vi "comm trail.vi"() -> ()   [LabVIEW 2017]
uses:
  <vilib>/NI/Modbus Library/API/Wrapper/Create TCP Master.vi
  <vilib>/NI/Modbus Library/API/master/Modbus Master.lvclass
  <vilib>/NI/Modbus Library/API/Wrapper/API Main.lvlib
panel:
  out "*(type *) &x":sgl
  out "*(type *) &x 2":sgl
  out "Converted Array":sgl[](array[numeric])
  out "register values 2":u16[](array[numeric])
  out "concatenated string":string
  out "ASCII VALUE":string[](array[string])
  out "discrete inputs":bool[](array[boolean])
  out "error out":errorcluster
  out "register values":u16[](array[numeric])
  out "coils":bool[](array[boolean])
  in  "stop":bool
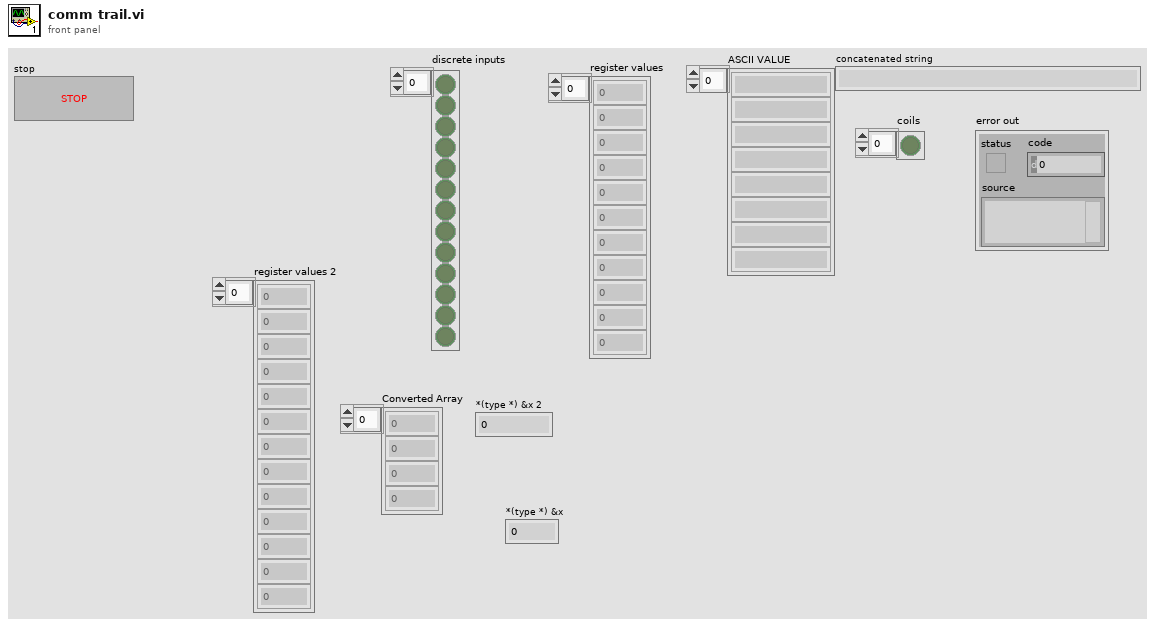
[diagram p1: front panel]
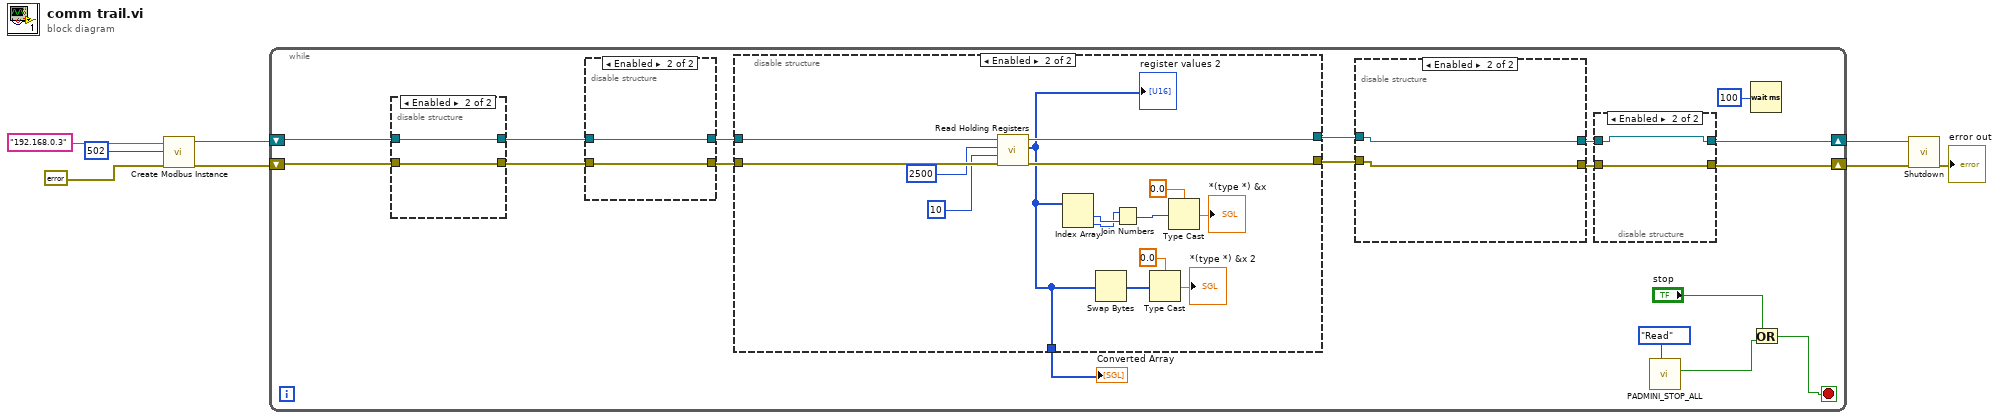
[diagram p0: block diagram]
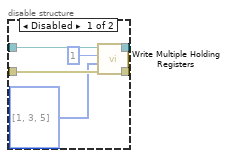
[diagram p2: hidden frame]
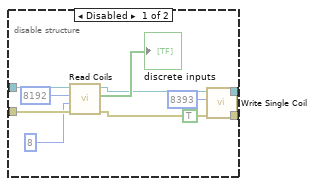
[diagram p3: hidden frame]
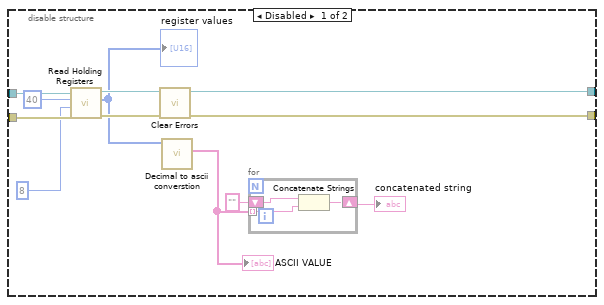
[diagram p4: hidden frame]
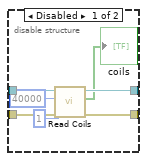
[diagram p5: hidden frame]
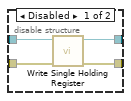
[diagram p6: hidden frame]
diagram:
  n1 = call-poly <vilib>:"Create Modbus Instance.vi"("error in"=errorcluster {"status"=FALSE, "code"=0, "source"=""}, "port (502)"=u16 502, "address"="192.168.0.3") -> ("error out"=w8:errorcluster, "TCP master instance"=w7:refnum<class "Modbus Master.lvclass">)  [unwired: 7 in]
  n2 = while {
    shift-right: [w12] -> w4
    shift-left: w7 -> [w26]
    shift-right: [w13] -> w5
    shift-left: w8 -> [w25]
    stop <- w22 stop-if-true
    n3 = disable-structure shown="Enabled" {
      disable-tunnel: w26 -> [w89 w91]
      disable-tunnel: w25 -> [w88 w90]
      disable-tunnel: [w87 w91] -> w20
      disable-tunnel: [w86 w90] -> w19
      frame Disabled {
        n4 = call-dynamic "Write Single Holding Register.vi"("error in"=w88, "Modbus master in"=w89) -> ("error out"=w86:errorcluster, "Modbus master out"=w87:refnum<class "Modbus Master.lvclass">)  [unwired: 8 in]
      }
      frame Enabled {
      }
    }
    n5 = disable-structure shown="Enabled" {
      disable-tunnel: w20 -> [w83 w85]
      disable-tunnel: w19 -> [w82 w84]
      disable-tunnel: [w81 w84] -> w18
      disable-tunnel: [w80 w85] -> w17
      frame Disabled {
        n6 = call-dynamic "Read Coils.vi"("error in"=w82, "number of inputs"=u16 1, "starting address"=u16 40000, "Modbus master in"=w83) -> ("error out"=w81:errorcluster, "coils"=→"coils":bool[], "Modbus master out"=w80:refnum<class "Modbus Master.lvclass">)  [unwired: 5 in]
      }
      frame Enabled {
      }
    }
    n7 = disable-structure shown="Enabled" {
      disable-tunnel: w18 -> [w58 w76]
      disable-tunnel: w17 -> [w57 w74]
      disable-tunnel: [w53 w73] -> w15
      disable-tunnel: [w52 w75] -> w14
      disable-tunnel: [_ w68] -> w9
      frame Disabled {
        n8 = call-dynamic "Read Holding Registers.vi"("error in"=w58, "number of inputs"=u16 8, "starting address"=u16 40, "Modbus master in"=w57) -> ("error out"=w54:errorcluster, "register values"=w51:u16[], "Modbus master out"=w53:refnum<class "Modbus Master.lvclass">)  [unwired: 5 in]
        "register values" <- w51
        n9 = call <vilib>:"Clear Errors.vi"("error in (no error)"=w54) -> ("error out"=w52:errorcluster)  [unwired: 5 in, 1 out]
        n10 = call "Decimal to ascii converstion.vi"("DECIMAL VALUE"=w51) -> ("ASCII VALUE"=w50:string[])  [unwired: 10 in]
        "ASCII VALUE" <- w50
        n11 = for {
          tunnel: w50 -> [w61] mode=indexing
          shift-right: [w60] -> w48
          shift-left: "" -> [w59]
          n12 = Concatenate Strings(w59, w61) -> (w60:string)
        }
        "concatenated string" <- w48
      }
      frame Enabled {
        n13 = call-dynamic "Read Holding Registers.vi"("error in"=w76, "number of inputs"=u16 10, "starting address"=u16 2500, "Modbus master in"=w74) -> ("error out"=w75:errorcluster, "register values"=w68:u16[], "Modbus master out"=w73:refnum<class "Modbus Master.lvclass">)  [unwired: 5 in]
        "register values 2" <- w68
        n14 = Index Array(array=w68) -> (element #1=w64:u16, element #2=w63:u16)  [unwired: 2 in]
        n15 = Swap Bytes(anything=w68) -> (byte swapped=w65:u16[])
        n16 = Join Numbers(hi=w63, lo=w64) -> ((hi.lo)=w69:u32)
        n17 = Type Cast(type=sgl 0.0, x=w65) -> (*(type *) &x=→"*(type *) &x 2":sgl)
        n18 = Type Cast(type=sgl 0.0, x=w69) -> (*(type *) &x=→"*(type *) &x":sgl)
      }
    }
    "Converted Array" <- w9
    n19 = disable-structure shown="Enabled" {
      disable-tunnel: w15 -> [w45 w47]
      disable-tunnel: w14 -> [w44 w46]
      disable-tunnel: [w39 w46] -> w11
      disable-tunnel: [w35 w47] -> w10
      frame Disabled {
        n20 = call-dynamic "Read Coils.vi"("error in"=w44, "number of inputs"=u16 8, "starting address"=u16 8192, "Modbus master in"=w45) -> ("error out"=w43:errorcluster, "coils"=→"discrete inputs":bool[], "Modbus master out"=w38:refnum<class "Modbus Master.lvclass">)  [unwired: 5 in]
        n21 = call-dynamic "Write Single Coil.vi"("error in"=w43, "coil to write"=TRUE, "address"=u16 8393, "Modbus master in"=w38) -> ("error out"=w39:errorcluster, "Modbus master out"=w35:refnum<class "Modbus Master.lvclass">)  [unwired: 6 in]
      }
      frame Enabled {
      }
    }
    n22 = disable-structure shown="Enabled" {
      disable-tunnel: [w32 w33] -> w13
      disable-tunnel: [w31 w34] -> w12
      disable-tunnel: w11 -> [w30 w33]
      disable-tunnel: w10 -> [w29 w34]
      frame Disabled {
        n23 = call-dynamic "Write Multiple Holding Registers.vi"("error in"=w30, "registers to write"=u16[] [1, 3, 5], "starting address"=u16 1, "Modbus master in"=w29) -> ("error out"=w32:errorcluster, "Modbus master out"=w31:refnum<class "Modbus Master.lvclass">)  [unwired: 6 in]
      }
      frame Enabled {
      }
    }
    n24 = call "PADMINI_STOP_ALL.vi"("Enum"=enum16{"Read", "Write"}."Read") -> ("Boolean 2"=w21:bool)  [unwired: 9 in, 1 out]
    n25 = Wait (ms)(milliseconds to wait=u32 100) -> ()  [unwired: 1 out]
    n26 = Or(x="stop", y=w21) -> (x .or. y?=w22:bool)
  }
  n27 = call-dynamic "Shutdown.vi"("error in"=w5, "Modbus master in"=w4) -> ("error out"=→"error out":errorcluster)  [unwired: 9 in]
